vi "Distend 3D Object.vi"(6 "Distend size":dbl, 9 "Distend method":T2=enum."Linear distance from center", 10 "Distend mode":T3, 11 "Normals and Coordinates":T1) -> (3 "Normals and Coordinates out":T1)   [LabVIEW 2015, in "Morph Cortical Surfaces.lvlib"]
doc: "Distend vertices by either distance from center of mass or by Normals. Balloon mode will change the size, Morph mode will keep the size of hemispheres."
uses:
  Morph Cortical Surfaces.lvlib
  Distend mode.ctl
  Distend method control.ctl
  Vertex data control.ctl
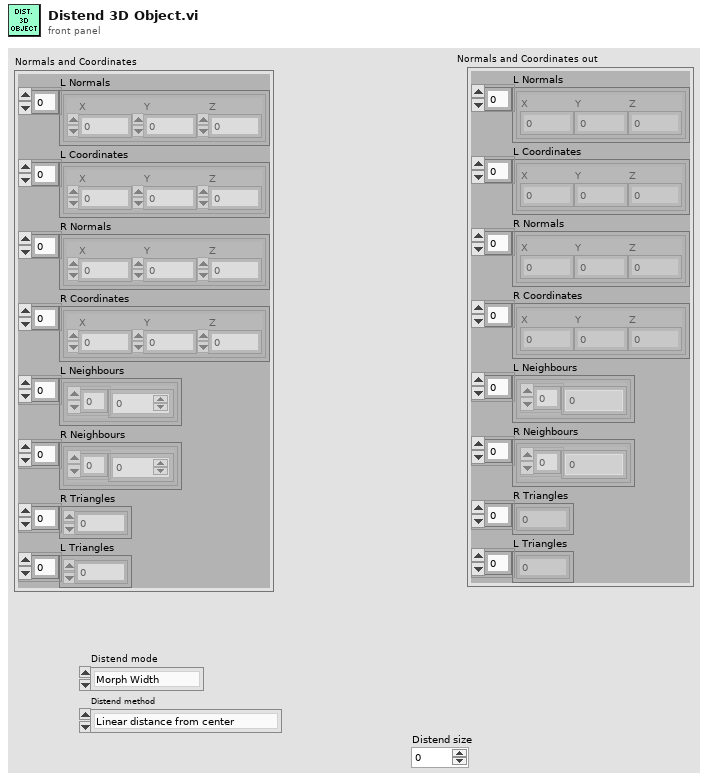
[diagram p1: front panel]
types:
  T1 = typedef "Morph Cortical Surfaces.lvlib/Vertex data control.ctl" = cluster{"L Normals":cluster{"X":sgl, "Y":sgl, "Z":sgl}[], "L Coordinates":cluster{"X":sgl, "Y":sgl, "Z":sgl}[], "R Normals":cluster{"X":sgl, "Y":sgl, "Z":sgl}[], "R Coordinates":cluster{"X":sgl, "Y":sgl, "Z":sgl}[], "L Neighbours":cluster{i32[]}[], "R Neighbours":cluster{i32[]}[], "R Triangles":i32[], "L Triangles":i32[]}
  T2 = typedef "Morph Cortical Surfaces.lvlib/Distend method control.ctl" = enum16{"Use weighting values", "Linear distance from center", "Exponential distance from center"}
  T3 = typedef "Morph Cortical Surfaces.lvlib/Distend mode.ctl" = enum16{"Morph Width", "Balloon Width", "Morph Height", "Balloon Height"}
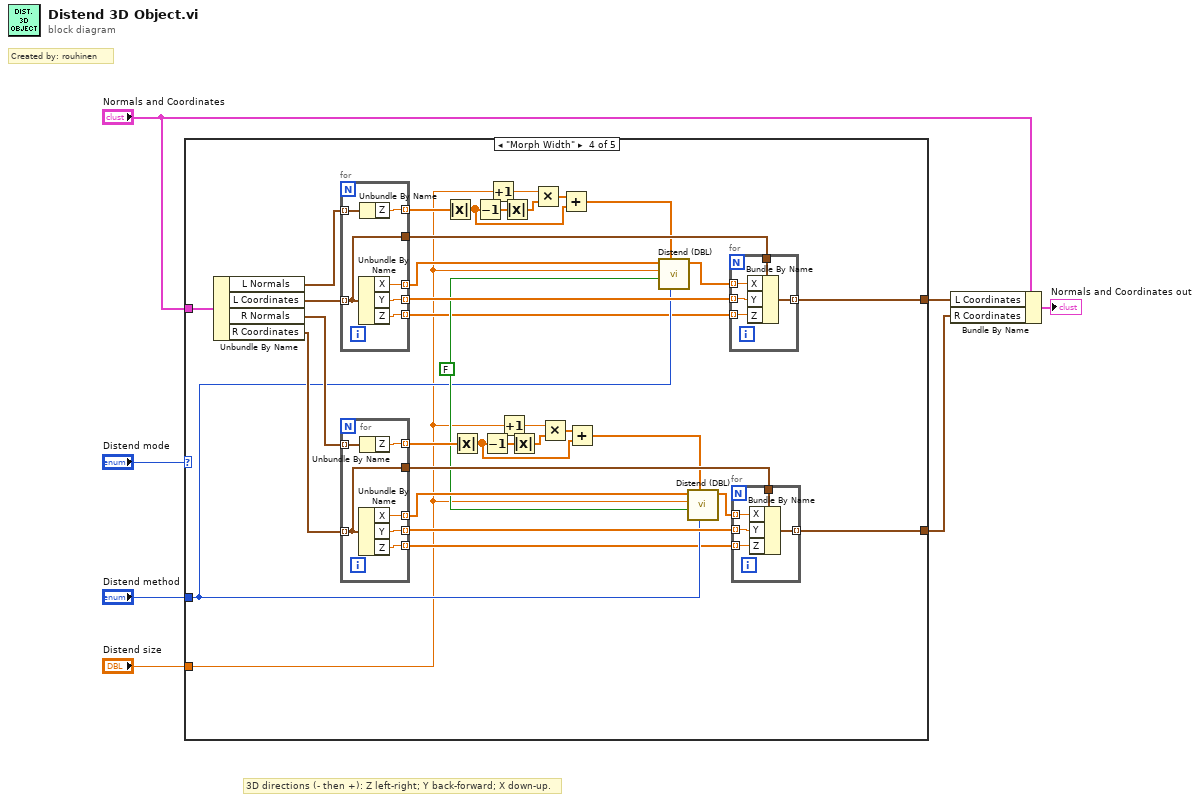
[diagram p0: block diagram]
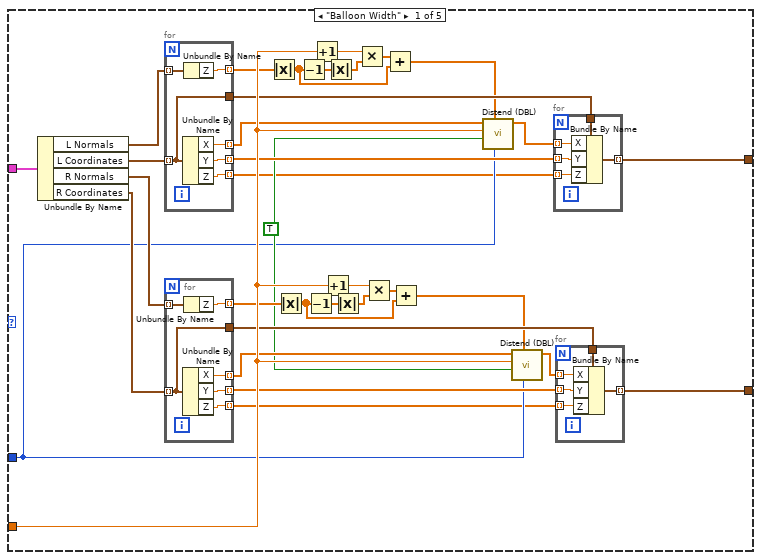
[diagram p2: hidden frame]
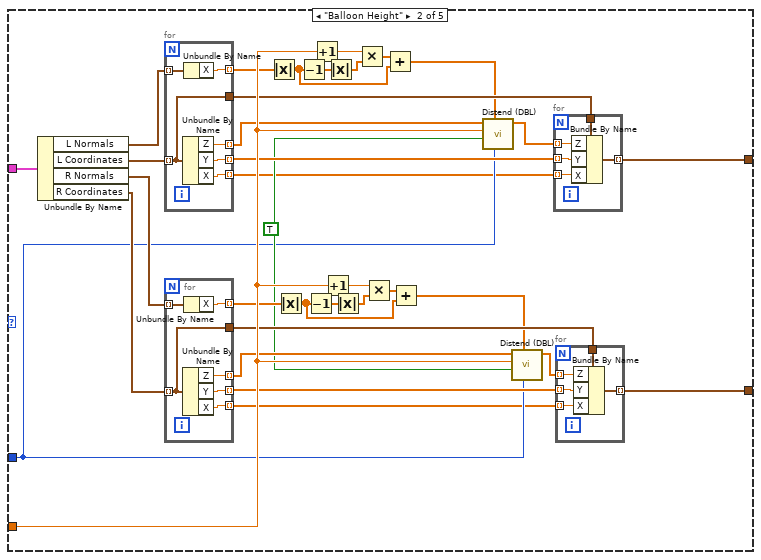
[diagram p3: hidden frame]
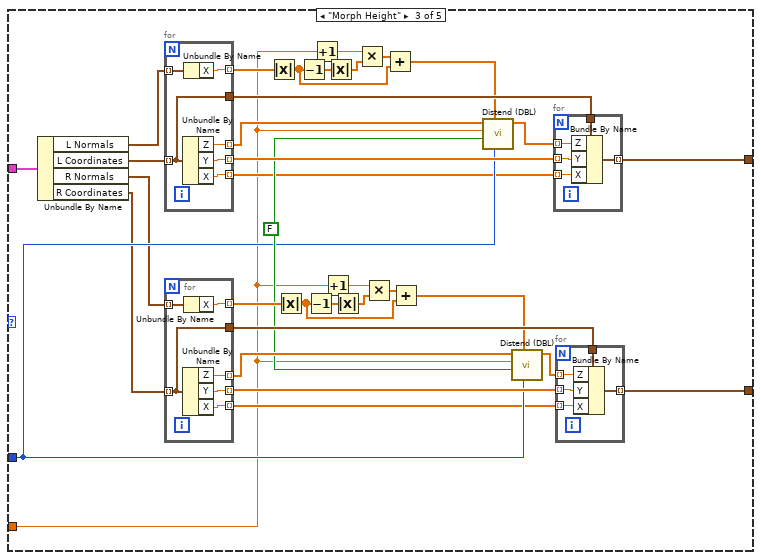
[diagram p4: hidden frame]
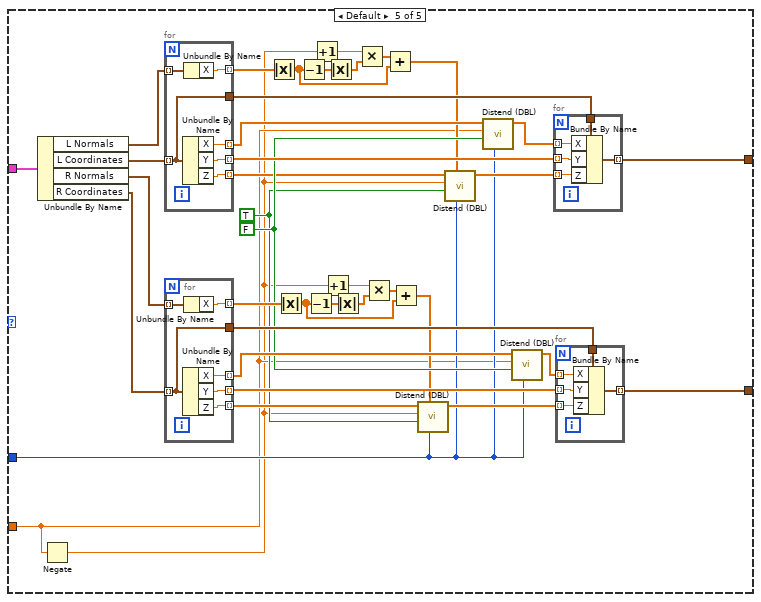
[diagram p5: hidden frame]
diagram:
  # "3D directions (- then +): Z left-right; Y back-forward; X down-up."
  # "Created by: rouhinen"
  n1 = case shown="\"Morph Width\"" "Distend mode" {
    tunnel: "Normals and Coordinates" -> [w39 w95 w153 w208 w268]
    tunnel: [w36 w92 w150 w205 w265] -> w7
    tunnel: [w31 w87 w145 w200 w258] -> w6
    tunnel: "Distend size" -> [w41 w97 w124 w176 w233]
    tunnel: "Distend method" -> [w12 w68 w129 w181 w234]
    frame "Balloon Width" {
      w18 = TRUE ("Keep silhuette size?(F)")
      n2 = Unbundle By Name(w39) -> ("L Normals"=w30:cluster{"X":sgl, "Y":sgl, "Z":sgl}[], "L Coordinates"=w40:cluster{"X":sgl, "Y":sgl, "Z":sgl}[], "R Normals"=w28:cluster{"X":sgl, "Y":sgl, "Z":sgl}[], "R Coordinates"=w29:cluster{"X":sgl, "Y":sgl, "Z":sgl}[])
      n3 = for {
        tunnel: w40 -> [w60] mode=indexing
        tunnel: [w63] -> w9 mode=indexing
        tunnel: [w62] -> w37 mode=indexing
        tunnel: [w61] -> w15 mode=indexing
        tunnel: [w60] -> w38
        tunnel: w30 -> [w59] mode=indexing
        tunnel: [w58] -> w14 mode=indexing
        n4 = Unbundle By Name(w60) -> ("X"=w61:sgl, "Y"=w62:sgl, "Z"=w63:sgl)
        n5 = Unbundle By Name(w59) -> ("Z"=w58:sgl)
      }
      n6 = for {
        tunnel: w29 -> [w49] mode=indexing
        tunnel: [w52] -> w11 mode=indexing
        tunnel: [w51] -> w34 mode=indexing
        tunnel: [w50] -> w32 mode=indexing
        tunnel: [w49] -> w33
        tunnel: w28 -> [w48] mode=indexing
        tunnel: [w47] -> w19 mode=indexing
        n7 = Unbundle By Name(w49) -> ("X"=w50:sgl, "Y"=w51:sgl, "Z"=w52:sgl)
        n8 = Unbundle By Name(w48) -> ("Z"=w47:sgl)
      }
      n9 = Absolute Value(x=w14) -> (abs(x)=w25:sgl[])
      n10 = Absolute Value(x=w19) -> (abs(x)=w23:sgl[])
      n11 = Decrement(x=w25) -> (x-1=w27:sgl[])
      n12 = Decrement(x=w23) -> (x-1=w20:sgl[])
      n13 = Increment(x=w41) -> (x+1=w16:dbl)
      n14 = Increment(x=w41) -> (x+1=w24:dbl)
      n15 = Absolute Value(x=w27) -> (abs(x)=w26:sgl[])
      n16 = Absolute Value(x=w20) -> (abs(x)=w22:sgl[])
      n17 = Multiply(x=w16, y=w26) -> (x*y=w17:dbl[])
      n18 = Multiply(x=w24, y=w22) -> (x*y=w21:dbl[])
      n19 = Add(x=w17, y=w25) -> (x+y=w10:dbl[])
      n20 = Add(x=w21, y=w23) -> (x+y=w8:dbl[])
      n21 = call "Distend (DBL).vi"("Distend method"=w12, "Weighting"=w10, "Keep silhuette size?(F)"=w18, "Distend"=w41, "X"=w15) -> ("X Distended"=w13:dbl[])  [unwired: 6 in]
      n22 = call "Distend (DBL).vi"("Distend method"=w12, "Weighting"=w8, "Keep silhuette size?(F)"=w18, "Distend"=w41, "X"=w32) -> ("X Distended"=w35:dbl[])  [unwired: 6 in]
      n23 = for {
        tunnel: w38 -> [w57]
        tunnel: w9 -> [w56] mode=indexing
        tunnel: w37 -> [w55] mode=indexing
        tunnel: w13 -> [w54] mode=indexing
        tunnel: [w53] -> w36 mode=indexing
        n24 = Bundle By Name(cluster=w57, "X"=w54, "Y"=w55, "Z"=w56) -> (w53:cluster{"X":sgl, "Y":sgl, "Z":sgl})
      }
      n25 = for {
        tunnel: w33 -> [w46]
        tunnel: w11 -> [w45] mode=indexing
        tunnel: w34 -> [w44] mode=indexing
        tunnel: w35 -> [w43] mode=indexing
        tunnel: [w42] -> w31 mode=indexing
        n26 = Bundle By Name(cluster=w46, "X"=w43, "Y"=w44, "Z"=w45) -> (w42:cluster{"X":sgl, "Y":sgl, "Z":sgl})
      }
    }
    frame "Balloon Height" {
      w74 = TRUE ("Keep silhuette size?(F)")
      n27 = Unbundle By Name(w95) -> ("L Normals"=w86:cluster{"X":sgl, "Y":sgl, "Z":sgl}[], "L Coordinates"=w96:cluster{"X":sgl, "Y":sgl, "Z":sgl}[], "R Normals"=w84:cluster{"X":sgl, "Y":sgl, "Z":sgl}[], "R Coordinates"=w85:cluster{"X":sgl, "Y":sgl, "Z":sgl}[])
      n28 = for {
        tunnel: w96 -> [w116] mode=indexing
        tunnel: [w119] -> w65 mode=indexing
        tunnel: [w118] -> w93 mode=indexing
        tunnel: [w117] -> w71 mode=indexing
        tunnel: [w116] -> w94
        tunnel: w86 -> [w115] mode=indexing
        tunnel: [w114] -> w70 mode=indexing
        n29 = Unbundle By Name(w116) -> ("Z"=w117:sgl, "Y"=w118:sgl, "X"=w119:sgl)
        n30 = Unbundle By Name(w115) -> ("X"=w114:sgl)
      }
      n31 = for {
        tunnel: w85 -> [w105] mode=indexing
        tunnel: [w108] -> w67 mode=indexing
        tunnel: [w107] -> w90 mode=indexing
        tunnel: [w106] -> w88 mode=indexing
        tunnel: [w105] -> w89
        tunnel: w84 -> [w104] mode=indexing
        tunnel: [w103] -> w75 mode=indexing
        n32 = Unbundle By Name(w105) -> ("Z"=w106:sgl, "Y"=w107:sgl, "X"=w108:sgl)
        n33 = Unbundle By Name(w104) -> ("X"=w103:sgl)
      }
      n34 = Absolute Value(x=w70) -> (abs(x)=w81:sgl[])
      n35 = Absolute Value(x=w75) -> (abs(x)=w79:sgl[])
      n36 = Decrement(x=w81) -> (x-1=w83:sgl[])
      n37 = Decrement(x=w79) -> (x-1=w76:sgl[])
      n38 = Increment(x=w97) -> (x+1=w72:dbl)
      n39 = Increment(x=w97) -> (x+1=w80:dbl)
      n40 = Absolute Value(x=w83) -> (abs(x)=w82:sgl[])
      n41 = Absolute Value(x=w76) -> (abs(x)=w78:sgl[])
      n42 = Multiply(x=w72, y=w82) -> (x*y=w73:dbl[])
      n43 = Multiply(x=w80, y=w78) -> (x*y=w77:dbl[])
      n44 = Add(x=w73, y=w81) -> (x+y=w66:dbl[])
      n45 = Add(x=w77, y=w79) -> (x+y=w64:dbl[])
      n46 = call "Distend (DBL).vi"("Distend method"=w68, "Weighting"=w66, "Keep silhuette size?(F)"=w74, "Distend"=w97, "X"=w71) -> ("X Distended"=w69:dbl[])  [unwired: 6 in]
      n47 = call "Distend (DBL).vi"("Distend method"=w68, "Weighting"=w64, "Keep silhuette size?(F)"=w74, "Distend"=w97, "X"=w88) -> ("X Distended"=w91:dbl[])  [unwired: 6 in]
      n48 = for {
        tunnel: w94 -> [w113]
        tunnel: w65 -> [w112] mode=indexing
        tunnel: w93 -> [w111] mode=indexing
        tunnel: w69 -> [w110] mode=indexing
        tunnel: [w109] -> w92 mode=indexing
        n49 = Bundle By Name(cluster=w113, "Z"=w110, "Y"=w111, "X"=w112) -> (w109:cluster{"X":sgl, "Y":sgl, "Z":sgl})
      }
      n50 = for {
        tunnel: w89 -> [w102]
        tunnel: w67 -> [w101] mode=indexing
        tunnel: w90 -> [w100] mode=indexing
        tunnel: w91 -> [w99] mode=indexing
        tunnel: [w98] -> w87 mode=indexing
        n51 = Bundle By Name(cluster=w102, "Z"=w99, "Y"=w100, "X"=w101) -> (w98:cluster{"X":sgl, "Y":sgl, "Z":sgl})
      }
    }
    frame "Morph Height" {
      w135 = FALSE ("Keep silhuette size?(F)")
      n52 = Unbundle By Name(w153) -> ("L Normals"=w120:cluster{"X":sgl, "Y":sgl, "Z":sgl}[], "L Coordinates"=w121:cluster{"X":sgl, "Y":sgl, "Z":sgl}[], "R Normals"=w122:cluster{"X":sgl, "Y":sgl, "Z":sgl}[], "R Coordinates"=w123:cluster{"X":sgl, "Y":sgl, "Z":sgl}[])
      n53 = for {
        tunnel: w121 -> [w172] mode=indexing
        tunnel: [w175] -> w126 mode=indexing
        tunnel: [w174] -> w151 mode=indexing
        tunnel: [w173] -> w132 mode=indexing
        tunnel: [w172] -> w152
        tunnel: w120 -> [w171] mode=indexing
        tunnel: [w170] -> w131 mode=indexing
        n54 = Unbundle By Name(w172) -> ("Z"=w173:sgl, "Y"=w174:sgl, "X"=w175:sgl)
        n55 = Unbundle By Name(w171) -> ("X"=w170:sgl)
      }
      n56 = for {
        tunnel: w123 -> [w161] mode=indexing
        tunnel: [w164] -> w128 mode=indexing
        tunnel: [w163] -> w148 mode=indexing
        tunnel: [w162] -> w146 mode=indexing
        tunnel: [w161] -> w147
        tunnel: w122 -> [w160] mode=indexing
        tunnel: [w159] -> w136 mode=indexing
        n57 = Unbundle By Name(w161) -> ("Z"=w162:sgl, "Y"=w163:sgl, "X"=w164:sgl)
        n58 = Unbundle By Name(w160) -> ("X"=w159:sgl)
      }
      n59 = Absolute Value(x=w131) -> (abs(x)=w142:sgl[])
      n60 = Absolute Value(x=w136) -> (abs(x)=w140:sgl[])
      n61 = Decrement(x=w142) -> (x-1=w144:sgl[])
      n62 = Decrement(x=w140) -> (x-1=w137:sgl[])
      n63 = Increment(x=w124) -> (x+1=w133:dbl)
      n64 = Increment(x=w124) -> (x+1=w141:dbl)
      n65 = Absolute Value(x=w144) -> (abs(x)=w143:sgl[])
      n66 = Absolute Value(x=w137) -> (abs(x)=w139:sgl[])
      n67 = Multiply(x=w133, y=w143) -> (x*y=w134:dbl[])
      n68 = Multiply(x=w141, y=w139) -> (x*y=w138:dbl[])
      n69 = Add(x=w134, y=w142) -> (x+y=w127:dbl[])
      n70 = Add(x=w138, y=w140) -> (x+y=w125:dbl[])
      n71 = call "Distend (DBL).vi"("Distend method"=w129, "Weighting"=w127, "Keep silhuette size?(F)"=w135, "Distend"=w124, "X"=w132) -> ("X Distended"=w130:dbl[])  [unwired: 6 in]
      n72 = call "Distend (DBL).vi"("Distend method"=w129, "Weighting"=w125, "Keep silhuette size?(F)"=w135, "Distend"=w124, "X"=w146) -> ("X Distended"=w149:dbl[])  [unwired: 6 in]
      n73 = for {
        tunnel: w152 -> [w169]
        tunnel: w126 -> [w168] mode=indexing
        tunnel: w151 -> [w167] mode=indexing
        tunnel: w130 -> [w166] mode=indexing
        tunnel: [w165] -> w150 mode=indexing
        n74 = Bundle By Name(cluster=w169, "Z"=w166, "Y"=w167, "X"=w168) -> (w165:cluster{"X":sgl, "Y":sgl, "Z":sgl})
      }
      n75 = for {
        tunnel: w147 -> [w158]
        tunnel: w128 -> [w157] mode=indexing
        tunnel: w148 -> [w156] mode=indexing
        tunnel: w149 -> [w155] mode=indexing
        tunnel: [w154] -> w145 mode=indexing
        n76 = Bundle By Name(cluster=w158, "Z"=w155, "Y"=w156, "X"=w157) -> (w154:cluster{"X":sgl, "Y":sgl, "Z":sgl})
      }
    }
    frame "Morph Width" {
      w187 = FALSE ("Keep silhuette size?(F)")
      n77 = Unbundle By Name(w208) -> ("L Normals"=w199:cluster{"X":sgl, "Y":sgl, "Z":sgl}[], "L Coordinates"=w209:cluster{"X":sgl, "Y":sgl, "Z":sgl}[], "R Normals"=w197:cluster{"X":sgl, "Y":sgl, "Z":sgl}[], "R Coordinates"=w198:cluster{"X":sgl, "Y":sgl, "Z":sgl}[])
      n78 = for {
        tunnel: w209 -> [w228] mode=indexing
        tunnel: [w231] -> w178 mode=indexing
        tunnel: [w230] -> w206 mode=indexing
        tunnel: [w229] -> w184 mode=indexing
        tunnel: [w228] -> w207
        tunnel: w199 -> [w227] mode=indexing
        tunnel: [w226] -> w183 mode=indexing
        n79 = Unbundle By Name(w228) -> ("X"=w229:sgl, "Y"=w230:sgl, "Z"=w231:sgl)
        n80 = Unbundle By Name(w227) -> ("Z"=w226:sgl)
      }
      n81 = for {
        tunnel: w198 -> [w217] mode=indexing
        tunnel: [w220] -> w180 mode=indexing
        tunnel: [w219] -> w203 mode=indexing
        tunnel: [w218] -> w201 mode=indexing
        tunnel: [w217] -> w202
        tunnel: w197 -> [w216] mode=indexing
        tunnel: [w215] -> w188 mode=indexing
        n82 = Unbundle By Name(w217) -> ("X"=w218:sgl, "Y"=w219:sgl, "Z"=w220:sgl)
        n83 = Unbundle By Name(w216) -> ("Z"=w215:sgl)
      }
      n84 = Absolute Value(x=w183) -> (abs(x)=w194:sgl[])
      n85 = Absolute Value(x=w188) -> (abs(x)=w192:sgl[])
      n86 = Decrement(x=w194) -> (x-1=w196:sgl[])
      n87 = Decrement(x=w192) -> (x-1=w189:sgl[])
      n88 = Increment(x=w176) -> (x+1=w185:dbl)
      n89 = Increment(x=w176) -> (x+1=w193:dbl)
      n90 = Absolute Value(x=w196) -> (abs(x)=w195:sgl[])
      n91 = Absolute Value(x=w189) -> (abs(x)=w191:sgl[])
      n92 = Multiply(x=w185, y=w195) -> (x*y=w186:dbl[])
      n93 = Multiply(x=w193, y=w191) -> (x*y=w190:dbl[])
      n94 = Add(x=w186, y=w194) -> (x+y=w179:dbl[])
      n95 = Add(x=w190, y=w192) -> (x+y=w177:dbl[])
      n96 = call "Distend (DBL).vi"("Distend method"=w181, "Weighting"=w179, "Keep silhuette size?(F)"=w187, "Distend"=w176, "X"=w184) -> ("X Distended"=w182:dbl[])  [unwired: 6 in]
      n97 = call "Distend (DBL).vi"("Distend method"=w181, "Weighting"=w177, "Keep silhuette size?(F)"=w187, "Distend"=w176, "X"=w201) -> ("X Distended"=w204:dbl[])  [unwired: 6 in]
      n98 = for {
        tunnel: w207 -> [w225]
        tunnel: w178 -> [w224] mode=indexing
        tunnel: w206 -> [w223] mode=indexing
        tunnel: w182 -> [w222] mode=indexing
        tunnel: [w221] -> w205 mode=indexing
        n99 = Bundle By Name(cluster=w225, "X"=w222, "Y"=w223, "Z"=w224) -> (w221:cluster{"X":sgl, "Y":sgl, "Z":sgl})
      }
      n100 = for {
        tunnel: w202 -> [w214]
        tunnel: w180 -> [w213] mode=indexing
        tunnel: w203 -> [w212] mode=indexing
        tunnel: w204 -> [w211] mode=indexing
        tunnel: [w210] -> w200 mode=indexing
        n101 = Bundle By Name(cluster=w214, "X"=w211, "Y"=w212, "Z"=w213) -> (w210:cluster{"X":sgl, "Y":sgl, "Z":sgl})
      }
    }
    frame Default {
      w245 = FALSE ("Keep silhuette size?(F)")
      w244 = TRUE ("Keep silhuette size?(F)")
      n102 = Unbundle By Name(w268) -> ("L Normals"=w257:cluster{"X":sgl, "Y":sgl, "Z":sgl}[], "L Coordinates"=w269:cluster{"X":sgl, "Y":sgl, "Z":sgl}[], "R Normals"=w255:cluster{"X":sgl, "Y":sgl, "Z":sgl}[], "R Coordinates"=w256:cluster{"X":sgl, "Y":sgl, "Z":sgl}[])
      n103 = Negate(x=w233) -> (-x=w232:dbl)
      n104 = for {
        tunnel: w269 -> [w288] mode=indexing
        tunnel: [w291] -> w240 mode=indexing
        tunnel: [w290] -> w266 mode=indexing
        tunnel: [w289] -> w241 mode=indexing
        tunnel: [w288] -> w267
        tunnel: w257 -> [w287] mode=indexing
        tunnel: [w286] -> w239 mode=indexing
        n105 = Unbundle By Name(w288) -> ("X"=w289:sgl, "Y"=w290:sgl, "Z"=w291:sgl)
        n106 = Unbundle By Name(w287) -> ("X"=w286:sgl)
      }
      n107 = for {
        tunnel: w256 -> [w277] mode=indexing
        tunnel: [w280] -> w259 mode=indexing
        tunnel: [w279] -> w263 mode=indexing
        tunnel: [w278] -> w260 mode=indexing
        tunnel: [w277] -> w261
        tunnel: w255 -> [w276] mode=indexing
        tunnel: [w275] -> w246 mode=indexing
        n108 = Unbundle By Name(w277) -> ("X"=w278:sgl, "Y"=w279:sgl, "Z"=w280:sgl)
        n109 = Unbundle By Name(w276) -> ("X"=w275:sgl)
      }
      n110 = Absolute Value(x=w239) -> (abs(x)=w252:sgl[])
      n111 = Absolute Value(x=w246) -> (abs(x)=w250:sgl[])
      n112 = Decrement(x=w252) -> (x-1=w254:sgl[])
      n113 = Decrement(x=w250) -> (x-1=w247:sgl[])
      n114 = Increment(x=w232) -> (x+1=w242:dbl)
      n115 = Increment(x=w232) -> (x+1=w251:dbl)
      n116 = Absolute Value(x=w254) -> (abs(x)=w253:sgl[])
      n117 = Absolute Value(x=w247) -> (abs(x)=w249:sgl[])
      n118 = Multiply(x=w242, y=w253) -> (x*y=w243:dbl[])
      n119 = Multiply(x=w251, y=w249) -> (x*y=w248:dbl[])
      n120 = Add(x=w243, y=w252) -> (x+y=w236:dbl[])
      n121 = Add(x=w248, y=w250) -> (x+y=w235:dbl[])
      n122 = call "Distend (DBL).vi"("Distend method"=w234, "Weighting"=w235, "Keep silhuette size?(F)"=w244, "Distend"=w232, "X"=w259) -> ("X Distended"=w262:dbl[])  [unwired: 6 in]
      n123 = call "Distend (DBL).vi"("Distend method"=w234, "Weighting"=w236, "Keep silhuette size?(F)"=w244, "Distend"=w232, "X"=w240) -> ("X Distended"=w238:dbl[])  [unwired: 6 in]
      n124 = call "Distend (DBL).vi"("Distend method"=w234, "Keep silhuette size?(F)"=w245, "Distend"=w233, "X"=w241) -> ("X Distended"=w237:dbl[])  [unwired: 7 in]
      n125 = call "Distend (DBL).vi"("Distend method"=w234, "Keep silhuette size?(F)"=w245, "Distend"=w233, "X"=w260) -> ("X Distended"=w264:dbl[])  [unwired: 7 in]
      n126 = for {
        tunnel: w267 -> [w285]
        tunnel: w238 -> [w284] mode=indexing
        tunnel: w266 -> [w283] mode=indexing
        tunnel: w237 -> [w282] mode=indexing
        tunnel: [w281] -> w265 mode=indexing
        n127 = Bundle By Name(cluster=w285, "X"=w282, "Y"=w283, "Z"=w284) -> (w281:cluster{"X":sgl, "Y":sgl, "Z":sgl})
      }
      n128 = for {
        tunnel: w261 -> [w274]
        tunnel: w262 -> [w273] mode=indexing
        tunnel: w263 -> [w272] mode=indexing
        tunnel: w264 -> [w271] mode=indexing
        tunnel: [w270] -> w258 mode=indexing
        n129 = Bundle By Name(cluster=w274, "X"=w271, "Y"=w272, "Z"=w273) -> (w270:cluster{"X":sgl, "Y":sgl, "Z":sgl})
      }
    }
  }
  n130 = Bundle By Name(cluster="Normals and Coordinates", "L Coordinates"=w7, "R Coordinates"=w6) -> (→"Normals and Coordinates out":T1)
